vi "Read Q.vi"(8 "error in (no error)":errorcluster, 11 "MC Data in":refnum<class "MC Data.lvclass">) -> (0 "error out":errorcluster, 2 "Q":sgl, 3 "MC Data out":refnum<class "MC Data.lvclass">)   [LabVIEW 2015, in "Alicat Lib.lvlib" / "MC Data.lvclass"]
uses:
  MC Data.lvclass
  MC Data.lvclass/MC Data.ctl
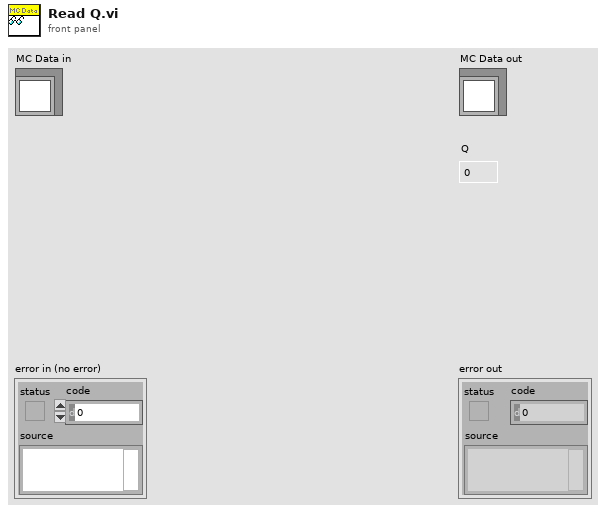
[diagram p1: front panel]
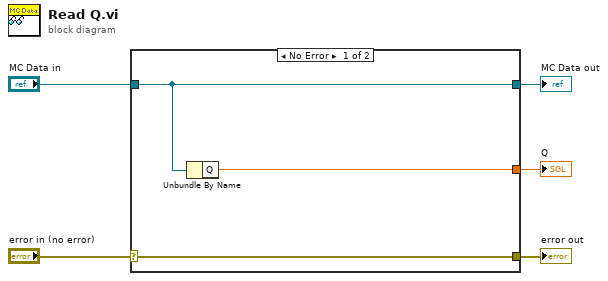
[diagram p0: block diagram]
diagram:
  n1 = case shown="No Error" "error in (no error)" {
    selector: "error in (no error)" -> [w8 w9]
    tunnel: [w8 w9] -> w4
    tunnel: [w7 w10] -> w2
    tunnel: "MC Data in" -> [w7 w10]
    tunnel: [w6 _] -> w1
    frame No Error {
      n2 = Unbundle By Name(w7) -> ("Q"=w6:sgl)
    }
    frame Error {
    }
  }
  "error out" <- w4
  "MC Data out" <- w2
  "Q" <- w1
